vi "Update DER_Measurement in Listbox.vi"(7 "DevIDs in Config":T1[](array[typedef]), 9 "Listbox Columns":T3, 10 "DER_Measurement (Array)":T2[](array[typedef]), 11 "MulticolumnListbox in":refnum<vi>) -> ()   [LabVIEW 2018, in "EMS User Interface Actor.lvlib" / "EMS User Interface.lvclass"]
uses:
  EMS User Interface.lvclass
  Controls/Listbox Columns.ctl
  <vilib>/ORNL/CSEISMIC DDS/CSEISMIC DDS Base/Data Types/DER_Measurement.ctl
  <vilib>/ORNL/CSEISMIC DDS/CSEISMIC DDS Base/Data Types/Controls/DeviceID.ctl
  <vilib>/Utility/miscctls.llb/LVRowAndColumnTypeDef.ctl
  <vilib>/Analysis/baseanly.llb/Mean (DBL).vi
  <vilib>/Analysis/NI_AALBase.lvlib
  <vilib>/ORNL/CSEISMIC DDS/CSEISMIC DDS Base/CSEISMIC DDS.lvclass
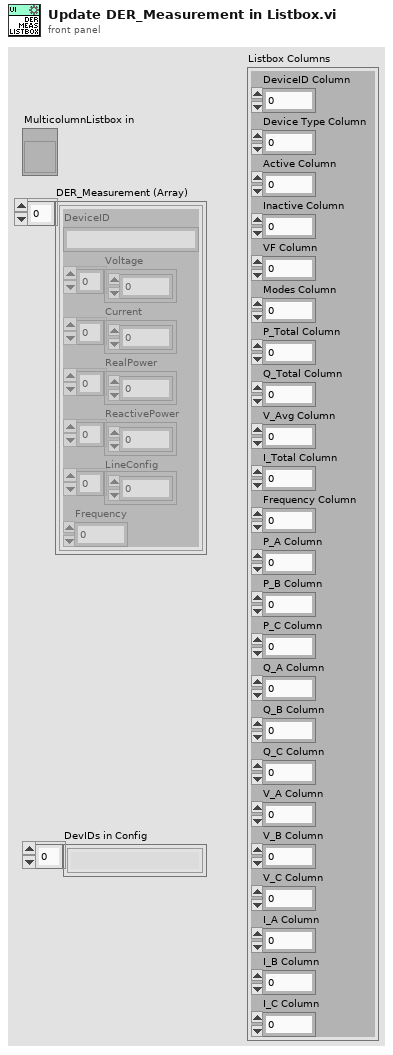
[diagram p1: front panel]
types:
  T1 = typedef "CSEISMIC DDS.lvlib/CSEISMIC DDS.lvclass/DeviceID.ctl" = string
  T2 = typedef "CSEISMIC DDS.lvlib/CSEISMIC DDS.lvclass/DER_Measurement.ctl" = cluster{"DeviceID":T1, "Voltage":dbl[], "Current":dbl[], "RealPower":dbl[], "ReactivePower":dbl[], "LineConfig":u8[], "Frequency":dbl}
  T3 = typedef "EMS User Interface Actor.lvlib/EMS User Interface.lvclass/Listbox Columns.ctl" = cluster{"DeviceID Column":i32, "Device Type Column":i32, "Active Column":i32, "Inactive Column":i32, "VF Column":i32, "Modes Column":i32, "P_Total Column":i32, "Q_Total Column":i32, "V_Avg Column":i32, "I_Total Column":i32, "Frequency Column":i32, "P_A Column":i32, "P_B Column":i32, "P_C Column":i32, "Q_A Column":i32, "Q_B Column":i32, "Q_C Column":i32, "V_A Column":i32, "V_B Column":i32, "V_C Column":i32, "I_A Column":i32, "I_B Column":i32, "I_C Column":i32}
  T4 = typedef "LVRowAndColumnTypeDef.ctl" = cluster{"Row":i32, "Column":i32}
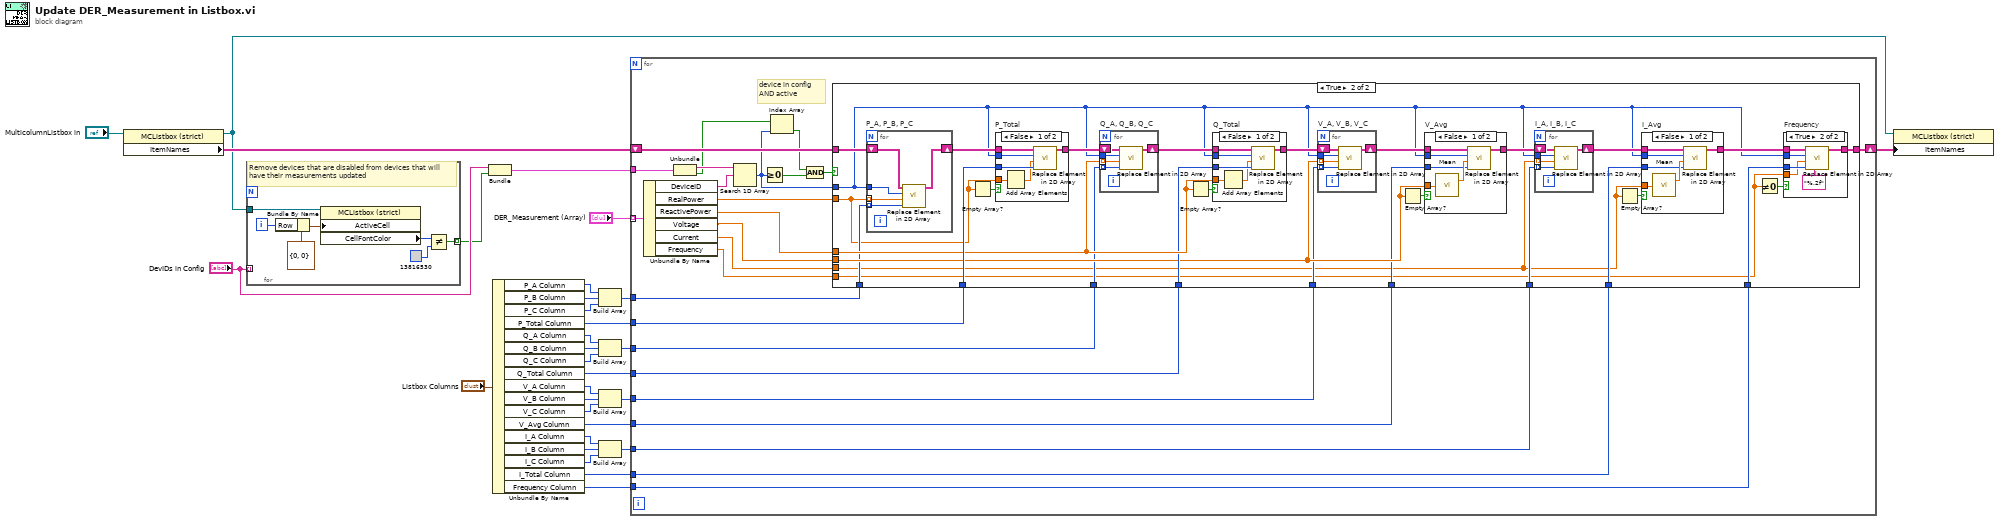
[diagram p0: block diagram]
diagram:
  n1 = property on="Property Node" class="MCListbox (strict)"(reference="MulticolumnListbox in") -> (reference out=w4:refnum<vi>, "ItemNames"=w5:string[][])  [unwired: 1 in, 1 out]
  n2 = for {
    tunnel: "DevIDs in Config" -> [_] mode=indexing
    tunnel: w4 -> [w37]
    tunnel: [w31] -> w2 mode=indexing
    i -> [w34]
    # "Remove devices that are disabled from devices that will have their measurements updated"
    n3 = Bundle By Name(cluster=T4 {"Row"=0, "Column"=0} ("Active Cell:Active Cell"), "Row"=w34) -> (w35:T4)
    n4 = property on="Property Node" class="MCListbox (strict)"(reference=w37, "ActiveCell"=w35) -> ("CellFontColor"=w33:u32)  [unwired: 1 in, 2 out]
    n5 = Not Equal?(x=w33, y=u32 13816530) -> (x != y?=w31:bool)
  }
  n6 = Bundle("DevIDs in Config"="DevIDs in Config", w2) -> (w1:cluster{"DevIDs in Config":T1[], bool[]})  [unwired: 1 in]
  n7 = Unbundle By Name("Listbox Columns") -> ("P_A Column"=w26:i32, "P_B Column"=w25:i32, "P_C Column"=w24:i32, "P_Total Column"=w28:i32, "Q_A Column"=w22:i32, "Q_B Column"=w21:i32, "Q_C Column"=w20:i32, "Q_Total Column"=w27:i32, "V_A Column"=w18:i32, "V_B Column"=w17:i32, "V_C Column"=w16:i32, "V_Avg Column"=w14:i32, "I_A Column"=w13:i32, "I_B Column"=w12:i32, "I_C Column"=w11:i32, "I_Total Column"=w9:i32, "Frequency Column"=w8:i32)
  n8 = Build Array(w26, w25, w24) -> (w23:i32[])
  n9 = Build Array(w22, w21, w20) -> (w19:i32[])
  n10 = Build Array(w18, w17, w16) -> (w15:i32[])
  n11 = Build Array(w13, w12, w11) -> (w10:i32[])
  n12 = for {
    tunnel: w1 -> [w62]
    tunnel: "DER_Measurement (Array)" -> [w61] mode=indexing
    tunnel: w28 -> [w58]
    tunnel: w27 -> [w56]
    tunnel: w15 -> [w52]
    tunnel: w23 -> [w54]
    tunnel: w19 -> [w53]
    tunnel: w14 -> [w51]
    tunnel: w10 -> [w50]
    tunnel: w9 -> [w49]
    tunnel: w8 -> [w47]
    shift-right: [w44] -> w6
    shift-left: w5 -> [w45]
    # "device in config AND active"
    n13 = Unbundle By Name(w61) -> ("DeviceID"=w60:T1, "RealPower"=w59:dbl[], "ReactivePower"=w57:dbl[], "Voltage"=w55:dbl[], "Current"=w48:dbl[], "Frequency"=w46:dbl)
    n14 = Unbundle(w62) -> ("DevIDs in Config"=w43:T1[], w40:bool[])
    n15 = Search 1D Array(1D array=w43, element=w60) -> (index of element=w39:i32)  [unwired: 1 in]
    n16 = Greater Or Equal To 0?(x=w39) -> (x >= 0?=w42:bool)
    n17 = Index Array(array=w40, index=w39) -> (element=w38:bool)
    n18 = Compound Arithmetic op=AND(w38, w42) -> (w41:bool)
    n19 = case shown="True" w41 {
      tunnel: w59 -> [_ w65]
      tunnel: w58 -> [_ w90]
      tunnel: w57 -> [_ w86]
      tunnel: w56 -> [_ w85]
      tunnel: w55 -> [_ w83]
      tunnel: w54 -> [_ w81]
      tunnel: w53 -> [_ w80]
      tunnel: w52 -> [_ w79]
      tunnel: w51 -> [_ w78]
      tunnel: w50 -> [_ w74]
      tunnel: w49 -> [_ w73]
      tunnel: w48 -> [_ w72]
      tunnel: w47 -> [_ w70]
      tunnel: w46 -> [_ w69]
      tunnel: w45 -> [w63 w67]
      tunnel: [w63 w66] -> w44
      tunnel: w39 -> [_ w64]
      frame False {
      }
      frame True {
        n20 = for "P_A, P_B, P_C" {
          tunnel: w81 -> [w102] mode=indexing
          tunnel: w65 -> [w103] mode=indexing
          shift-right: [w104] -> w93
          shift-left: w67 -> [w105]
          tunnel: w64 -> [w101]
          # "P_A, P_B, and P_C"
          n21 = call "Replace Element in 2D Array.vi"("Column"=w102, "Value"=w103, "Row"=w101, "ItemNames in"=w105) -> ("ItemNames out"=w104:string[][])  [unwired: 7 in]
        }
        n22 = Empty Array?(array=w65) -> (empty?=w92:bool)
        n23 = case "P_Total" shown="False" w92 {
          tunnel: w93 -> [w108 w112]
          tunnel: w65 -> [w111 _]
          tunnel: [w106 w112] -> w89
          tunnel: w64 -> [w107 _]
          tunnel: w90 -> [w110 _]
          frame False {
            n24 = Add Array Elements(numeric array=w111) -> (sum=w109:dbl)
            n25 = call "Replace Element in 2D Array.vi"("Column"=w110, "Value"=w109, "Row"=w107, "ItemNames in"=w108) -> ("ItemNames out"=w106:string[][])  [unwired: 7 in]
          }
          frame True {
          }
        }
        n26 = for "Q_A, Q_B, Q_C" {
          tunnel: w64 -> [w129]
          tunnel: w80 -> [w125] mode=indexing
          tunnel: w86 -> [w126] mode=indexing
          shift-right: [w127] -> w87
          shift-left: w89 -> [w128]
          # "P_A, P_B, and P_C"
          n27 = call "Replace Element in 2D Array.vi"("Column"=w125, "Value"=w126, "Row"=w129, "ItemNames in"=w128) -> ("ItemNames out"=w127:string[][])  [unwired: 7 in]
        }
        n28 = Empty Array?(array=w86) -> (empty?=w88:bool)
        n29 = case "Q_Total" shown="False" w88 {
          tunnel: w87 -> [w132 w136]
          tunnel: w86 -> [w135 _]
          tunnel: [w130 w136] -> w84
          tunnel: w64 -> [w131 _]
          tunnel: w85 -> [w134 _]
          frame False {
            n30 = Add Array Elements(numeric array=w135) -> (sum=w133:dbl)
            n31 = call "Replace Element in 2D Array.vi"("Column"=w134, "Value"=w133, "Row"=w131, "ItemNames in"=w132) -> ("ItemNames out"=w130:string[][])  [unwired: 7 in]
          }
          frame True {
          }
        }
        n32 = for "V_A, V_B, V_C" {
          tunnel: w64 -> [w141]
          tunnel: w79 -> [w137] mode=indexing
          tunnel: w83 -> [w138] mode=indexing
          shift-right: [w139] -> w82
          shift-left: w84 -> [w140]
          # "P_A, P_B, and P_C"
          n33 = call "Replace Element in 2D Array.vi"("Column"=w137, "Value"=w138, "Row"=w141, "ItemNames in"=w140) -> ("ItemNames out"=w139:string[][])  [unwired: 7 in]
        }
        n34 = Empty Array?(array=w83) -> (empty?=w91:bool)
        n35 = case "V_Avg" shown="False" w91 {
          tunnel: w82 -> [w145 w148]
          tunnel: w83 -> [w147 _]
          tunnel: [w142 w148] -> w75
          tunnel: w64 -> [w144 _]
          tunnel: w78 -> [w143 _]
          frame False {
            n36 = call-poly <vilib>:"Mean.vi"("X"=w147) -> ("mean"=w146:dbl)  [unwired: 1 out]
            n37 = call "Replace Element in 2D Array.vi"("Column"=w143, "Value"=w146, "Row"=w144, "ItemNames in"=w145) -> ("ItemNames out"=w142:string[][])  [unwired: 7 in]
          }
          frame True {
          }
        }
        n38 = for "I_A, I_B, I_C" {
          tunnel: w64 -> [w117]
          tunnel: w74 -> [w113] mode=indexing
          tunnel: w72 -> [w114] mode=indexing
          shift-right: [w115] -> w77
          shift-left: w75 -> [w116]
          # "P_A, P_B, and P_C"
          n39 = call "Replace Element in 2D Array.vi"("Column"=w113, "Value"=w114, "Row"=w117, "ItemNames in"=w116) -> ("ItemNames out"=w115:string[][])  [unwired: 7 in]
        }
        n40 = Empty Array?(array=w72) -> (empty?=w76:bool)
        n41 = case "I_Avg" shown="False" w76 {
          tunnel: w77 -> [w121 w124]
          tunnel: w72 -> [w123 _]
          tunnel: [w118 w124] -> w71
          tunnel: w64 -> [w120 _]
          tunnel: w73 -> [w119 _]
          frame False {
            n42 = call-poly <vilib>:"Mean.vi"("X"=w123) -> ("mean"=w122:dbl)  [unwired: 1 out]
            n43 = call "Replace Element in 2D Array.vi"("Column"=w119, "Value"=w122, "Row"=w120, "ItemNames in"=w121) -> ("ItemNames out"=w118:string[][])  [unwired: 7 in]
          }
          frame True {
          }
        }
        n44 = Not Equal To 0?(x=w69) -> (x != 0?=w68:bool)
        n45 = case "Frequency" shown="True" w68 {
          tunnel: w71 -> [w94 w100]
          tunnel: [w94 w99] -> w66
          tunnel: w64 -> [_ w98]
          tunnel: w70 -> [_ w97]
          tunnel: w69 -> [_ w96]
          frame False {
          }
          frame True {
            n46 = call "Replace Element in 2D Array.vi"("format string (%d)"="%.2f", "Column"=w97, "Value"=w96, "Row"=w98, "ItemNames in"=w100) -> ("ItemNames out"=w99:string[][])  [unwired: 6 in]
          }
        }
      }
    }
  }
  n47 = property on="Property Node" class="MCListbox (strict)"(reference=w4, "ItemNames"=w6) -> ()  [unwired: 1 in, 2 out]
